vi "Build Tree View.vi"(0 "Root Directory":string, 1 "Directory Tree in":T1, 2 "TreeControl in":refnum<vi>) -> ()   [LabVIEW 2020, in "AoC 2022.lvlib"]
uses:
  AoC 2022.lvlib
  Directory Tree.ctl
  Directory Contents.ctl
  File.ctl
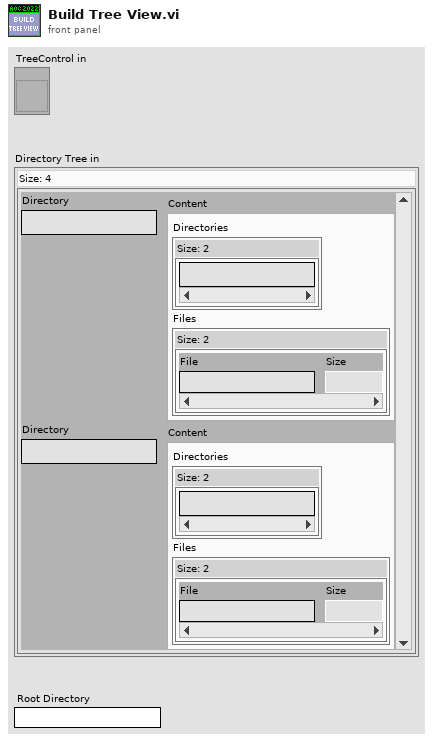
[diagram p1: front panel]
types:
  T1 = typedef "AoC 2022.lvlib/Directory Tree.ctl" = map{string, T2}
  T2 = typedef "AoC 2022.lvlib/Directory Contents.ctl" = cluster{"Directories":set{string}, "Files":T3}
  T3 = typedef "AoC 2022.lvlib/File.ctl" = map{string, u64}
  T4 = cluster{"Left Cell String":string, "Child Text":string[], "Child Tag":string, "Item Indent":i32, "Child Only?":bool, "Glyph Index":i32}[]
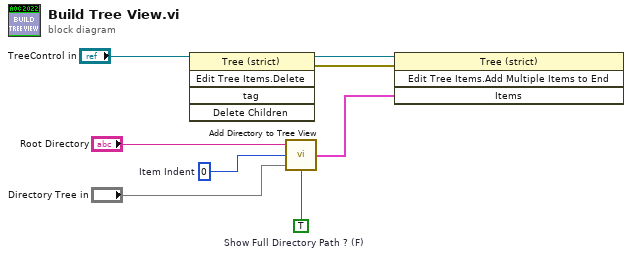
[diagram p0: block diagram]
diagram:
  w1 = TRUE  # Show Full Directory Path ? (F)
  w3 = 0  # Item Indent
  n1 = invoke class="Tree (strict)" method="Edit Tree Items.Delete"(reference="TreeControl in") -> (reference out=w7:refnum<vi>, error out=w8:errorcluster)  [unwired: 4 in, 3 out]
  n2 = call "Add Directory to Tree View.vi"("Show Full Directory Path ? (F)"=w1, "Directory Tree in"="Directory Tree in", "Item Indent"=w3, "Directory"="Root Directory") -> ("Tree View"=w2:T4)
  n3 = invoke class="Tree (strict)" method="Edit Tree Items.Add Multiple Items to End"(reference=w7, error in=w8, "Items"=w2) -> ()  [unwired: 1 in, 4 out]
